vi "FGV_Data.vi"(8 "error in (no error)":errorcluster, 10 "Option":T1=enum."Set", 11 "Data In":T2={"IMAQdx Session"="", "Resampled Image"=refnum, "Low Level Grab"=refnum, "X Resolution"=0, "Y Resolution"=0, "Image Threshold"=0, "Reset Value"=0, "FIFO Timer"=0, "Row Timer"=0, "Memory Writer Timer"=0, "Color"=enum."Red", "Top"=array32x96[3072 elements], "Bottom"=array32x96[3072 elements], "Timeout (ms)"=0, "Menu Tag"="", "Color Background"=enum."White", "FPGA VI Reference"=refnum, "Next Steps"=[], "Turn off LED Matrix"=FALSE, "FPGA Alias"="", "FPGA Bitfile"=path "", "Localized Texts"={"Status Text"={"Status Text Table"=[], "Status Text Index"=0}, "Controls"={"Control Text Table"=[], "Control Text Index"=0}, "Titles"={"Titles Text Table"=[], "Titles Text Index"=0}}, "Language"=0} {"Language" items=["English", "Español", "Português"]}) -> (0 "error out":errorcluster, 3 "Data Out":T2={"IMAQdx Session"="", "Resampled Image"=refnum, "Low Level Grab"=refnum, "X Resolution"=0, "Y Resolution"=0, "Image Threshold"=0, "Reset Value"=0, "FIFO Timer"=0, "Row Timer"=0, "Memory Writer Timer"=0, "Color"=enum."Red", "Top"=array32x96[3072 elements], "Bottom"=array32x96[3072 elements], "Timeout (ms)"=0, "Menu Tag"="", "Color Background"=enum."White", "FPGA VI Reference"=refnum, "Next Steps"=[], "Turn off LED Matrix"=FALSE, "FPGA Alias"="", "FPGA Bitfile"=path "", "Localized Texts"={"Status Text"={"Status Text Table"=[], "Status Text Index"=0}, "Controls"={"Control Text Table"=[], "Control Text Index"=0}, "Titles"={"Titles Text Table"=[], "Titles Text Index"=0}}, "Language"=0} {"Language" items=["English", "Español", "Português"]})   [LabVIEW 2015]
uses:
  Controls/HID Data.ctl
  <vilib>/userdefined/High Color/IMAQdx.ctl
  <vilib>/vision/Image Controls.llb/IMAQ Image.ctl
  Controls/HID State.ctl
  Controls/FGV_Options.ctl
  <vilib>/Utility/xml.llb/Read From XML File(string).vi
  <vilib>/Utility/xml.llb/Write to XML File(string).vi
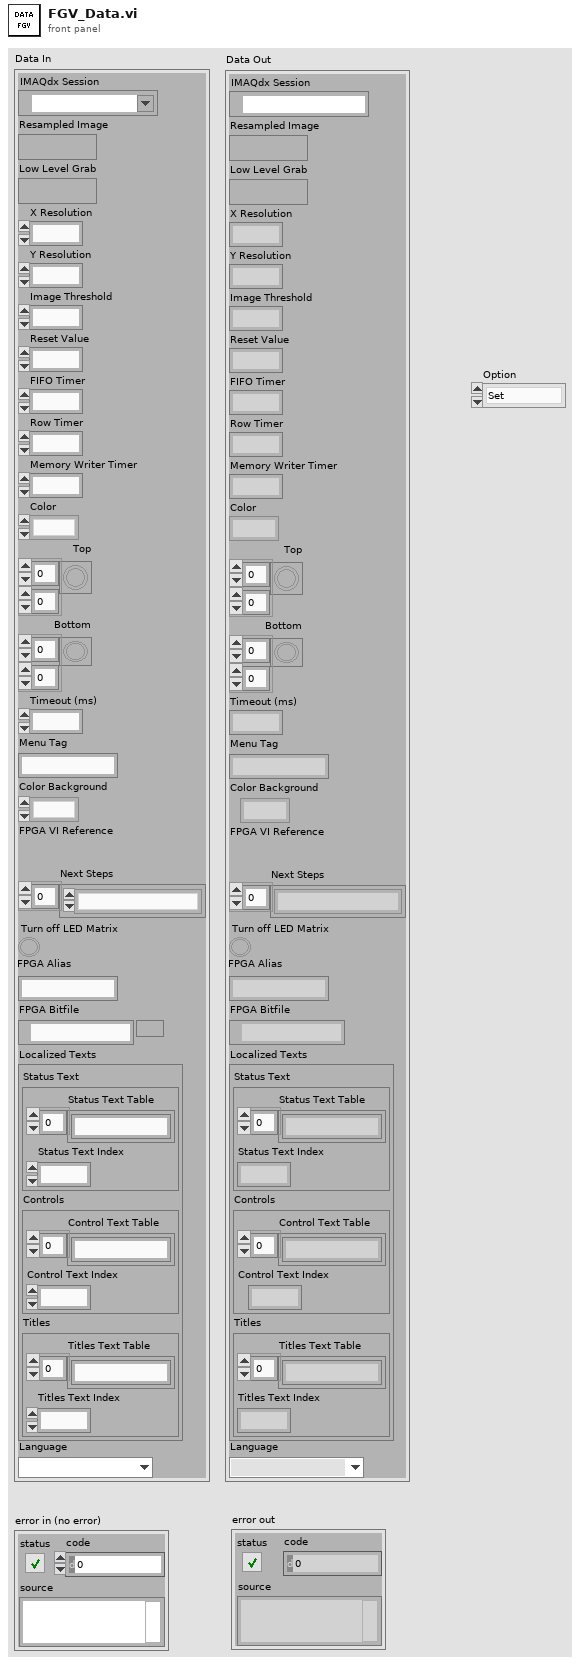
[diagram p1: front panel]
types:
  T1 = typedef "FGV_Options.ctl" = enum16{"Read from File", "Write to File", "Get", "Set"}
  T2 = typedef "HID Data.ctl" = cluster{"IMAQdx Session":T3, "Resampled Image":T4, "Low Level Grab":T4, "X Resolution":i32, "Y Resolution":i32, "Image Threshold":u8, "Reset Value":i32, "FIFO Timer":u16, "Row Timer":u32, "Memory Writer Timer":u8, "Color":enum16{"Green", "Blue", "Red", "White", "Pink", "Yellow", "Turquoise", "Black"}, "Top":bool[][], "Bottom":bool[][], "Timeout (ms)":i32, "Menu Tag":string, "Color Background":enum16{"Green", "Blue", "Red", "White", "Pink", "Yellow", "Turquoise", "Black"}, "FPGA VI Reference":refnum<k20>, "Next Steps":T5[], "Turn off LED Matrix":bool, "FPGA Alias":string, "FPGA Bitfile":path, "Localized Texts":cluster{"Status Text":cluster{"Status Text Table":string[], "Status Text Index":i32}, "Controls":cluster{"Control Text Table":string[], "Control Text Index":i32}, "Titles":cluster{"Titles Text Table":string[], "Titles Text Index":i32}}, "Language":u16}
  T3 = typedef "IMAQdx.ctl" = refnum<k21>
  T4 = typedef "IMAQ Image.ctl" = refnum<image>
  T5 = typedef "HID State.ctl" = enum16{"Initialize", "Set FPGA Parametes", "Set Camera Parameters", "Set LED Matrix Parameters", "Initialize FPGA Interface", "Initialize Camera", "Start FPGA VI", "Start Camera", "Wait for Event", "Update UI", "Acquire", "Process Image", "Get Boolean Arrays", "Send to FPGA", "Menu Pop-Up", "Menu Actions", "Handle Errors", "Close Camera", "Close FPGA", "Stop", "Exit"}
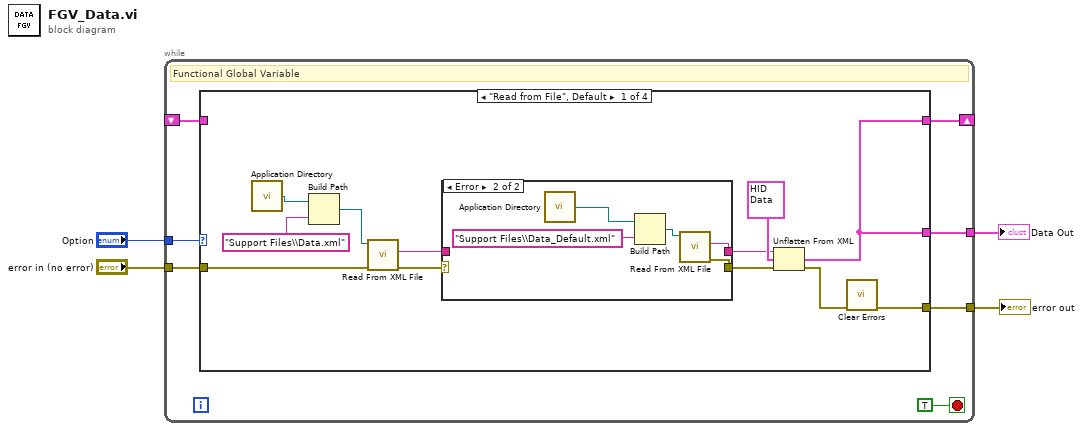
[diagram p0: block diagram]
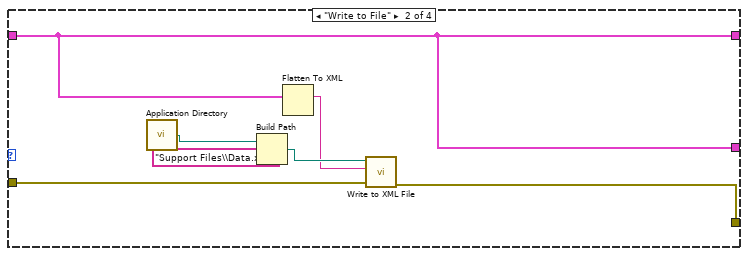
[diagram p3: hidden frame]
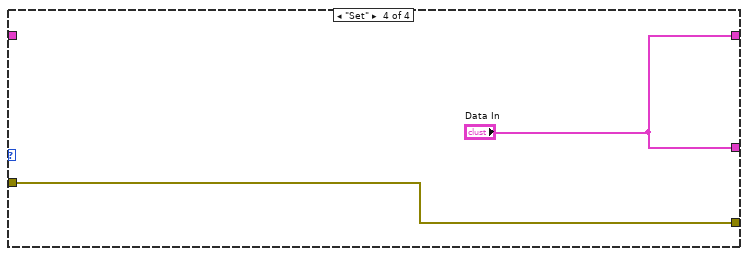
[diagram p5: hidden frame]
diagram:
  n1 = while {
    tunnel: "Option" -> [w11]
    shift-right: [w10] -> _
    shift-left: _ -> [w9]
    tunnel: [w8] -> w3
    tunnel: "error in (no error)" -> [w6]
    tunnel: [w5] -> w1
    stop <- TRUE stop-if-true
    # "Functional Global Variable"
    n2 = case shown="\"Read from File\", Default" w11 {
      tunnel: [w20 w35 w39 "Data In"] -> w10
      tunnel: w9 -> [_ w35 w39 _]
      tunnel: [w20 w35 w39 "Data In"] -> w8
      tunnel: w6 -> [w17 w32 w38 w40]
      tunnel: [w19 w31 w38 w40] -> w5
      frame "Read from File", Default {
        n3 = call <vilib>:"Application Directory.vi"() -> ("Application Directory"=w23:path)
        n4 = Build Path(base path=w23, name or relative path="Support Files\\Data.xml") -> (appended path=w18:path)
        n5 = call-poly <vilib>:"Read From XML File.vi"("error in (no error)"=w17, "XML File Path"=w18) -> ("error out"=w15:errorcluster, "XML Elements"=w14:string)  [unwired: 7 in, 1 out]
        n6 = case shown="Error" w15 {
          selector: w15 -> [w24 _]
          tunnel: w14 -> [w25 _]
          tunnel: [w25 w27] -> w13
          tunnel: [w24 w28] -> w12
          frame No Error {
          }
          frame Error {
            n7 = call <vilib>:"Application Directory.vi"() -> ("Application Directory"=w29:path)
            n8 = Build Path(base path=w29, name or relative path="Support Files\\Data_Default.xml") -> (appended path=w26:path)
            n9 = call-poly <vilib>:"Read From XML File.vi"("XML File Path"=w26) -> ("error out"=w28:errorcluster, "XML Elements"=w27:string)  [unwired: 8 in, 1 out]
          }
        }
        n10 = Unflatten From XML(xml string=w13, type=T2 {"IMAQdx Session"="", "Resampled Image"=refnum, "Low Level Grab"=refnum, "X Resolution"=0, "Y Resolution"=0, "Image Threshold"=0, "Reset Value"=0, "FIFO Timer"=0, "Row Timer"=0, "Memory Writer Timer"=0, "Color"=enum."Blue", "Top"=[], "Bottom"=[], "Timeout (ms)"=0, "Menu Tag"="", "Color Background"=enum."White", "FPGA VI Reference"=refnum, "Next Steps"=[enum."Wait for Event"], "Turn off LED Matrix"=FALSE, "FPGA Alias"="", "FPGA Bitfile"=path "", "Localized Texts"={"Status Text"={"Status Text Table"=[], "Status Text Index"=0}, "Controls"={"Control Text Table"=[], "Control Text Index"=0}, "Titles"={"Titles Text Table"=[], "Titles Text Index"=0}}, "Language"=0} ("Data Out"), error in (no error)=w12) -> (value=w20:T2, error out=w16:errorcluster)
        n11 = call <vilib>:"Clear Errors.vi"("error in (no error)"=w16) -> ("error out"=w19:errorcluster)  [unwired: 5 in, 1 out]
      }
      frame "Write to File" {
        n12 = call <vilib>:"Application Directory.vi"() -> ("Application Directory"=w37:path)
        n13 = Build Path(base path=w37, name or relative path="Support Files\\Data.xml") -> (appended path=w34:path)
        n14 = Flatten To XML(anything=w35) -> (xml string=w33:string)
        n15 = call-poly <vilib>:"Write to XML File.vi"("error in (no error)"=w32, "XML Input"=w33, "XML File Path"=w34) -> ("error out"=w31:errorcluster)  [unwired: 6 in, 2 out]
      }
      frame "Get" {
      }
      frame "Set" {
      }
    }
  }
  "Data Out" <- w3
  "error out" <- w1
